vi "MGI RWA Get Type Info.vi"(8 "Error In":errorcluster, 11 "Variant":variant) -> (0 "Error Out":errorcluster, 2 "Name":string, 3 "Type Enum":T1)   [LabVIEW 2018]
doc: "Return information about the datatype stored in Variant.\nType Enum is the type of data\nName is the name of the data\nIf the data is defined by a Type Definition, HasTypedef is true and Typedef contains information about the Type Definition.\n\nNote: This VI is similar to vi.lib/Utility/VariantDataType/GetTypeInfo.vi, and produces the exact same results, but this VI is much faster for Waveform Types. (For 4000 Waveform type elements, this VI takes around 8000 ms and the vi.lib takes around 1600 ms. \n\nAuthored by Robert C. Mortensen\nsupport@mooregoodideas.com\nwww.mooregoodideas.com\n\nCopyright (c) 2010, Moore Good Ideas, Inc.\n\nAll rights reserved.\n\nRedistribution and use in source and binary forms, with or without modification, are permitted provided that the following conditions are met:\n\n * Redistributions of source code must retain the above copyright notice, this list of conditions and the following disclaimer.\n * Redistributions in binary form must reproduce the above copyright notice, this list of conditions and the following disclaimer in the documentation and/or other materials provided with the distribution.\n * Neither the name of Moore Good Ideas, Inc. nor the names of its contributors may be used to endorse or promote products derived from this software without specific prior written permission.\n\nTHIS SOFTWARE IS PROVIDED BY THE COPYRIGHT HOLDERS AND CONTRIBUTORS \"AS IS\" AND ANY EXPRESS OR IMPLIED WARRANTIES, INCLUDING, BUT NOT LIMITED TO, THE IMPLIED WARRANTIES OF MERCHANTABILITY AND FITNESS FOR A PARTICULAR PURPOSE ARE DISCLAIMED. IN NO EVENT SHALL THE COPYRIGHT OWNER OR CONTRIBUTORS BE LIABLE FOR ANY DIRECT, INDIRECT, INCIDENTAL, SPECIAL, EXEMPLARY, OR CONSEQUENTIAL DAMAGES (INCLUDING, BUT NOT LIMITED TO, PROCUREMENT OF SUBSTITUTE GOODS OR SERVICES; LOSS OF USE, DATA, OR PROFITS; OR BUSINESS INTERRUPTION) HOWEVER CAUSED AND ON ANY THEORY OF LIABILITY, WHETHER IN CONTRACT, STRICT LIABILITY, OR TORT (INCLUDING NEGLIGENCE OR OTHERWISE) ARISING IN ANY WAY OUT OF THE USE OF THIS SOFTWARE, EVEN IF ADVISED OF THE POSSIBILITY OF SUCH DAMAGE."
uses:
  Type.ctl
  TypedefInfo.ctl
  VariantType.lvlib
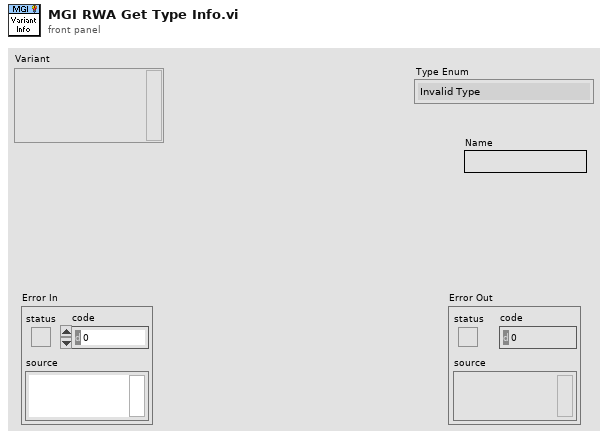
[diagram p1: front panel]
types:
  T1 = typedef "VariantType.lvlib/Type.ctl" = enum8{"Invalid Type", "Void", "I8", "I16", "I32", "I64", "U8", "U16", "U32", "U64", "Single Float", "Double Float", "Extended Float", "Single Complex", "Double Complex", "Extended Complex", "Enum U8", "Enum U16", "Enum U32", "Enum U64", "Single Float With Unit", "Double Float With Unit", "Extended Float With Unit", "Single Complex with Unit", "Double Complex with Unit", "Extended Complex with Unit", "Boolean", "String", "Path", "Picture", "Tag", "Array", "Cluster", "Variant", "LV Variant", "Waveform", "Timestamp", "Digital Waveform", "Digital Data", "ExpressData", "Refnum", "External Data", "VI", "Poly VI", "LabVIEW Class Instance", "Fixed Point"}
  T2 = typedef "VariantType.lvlib/TypedefInfo.ctl" = cluster{"Name":string, "Timestamp":u32}
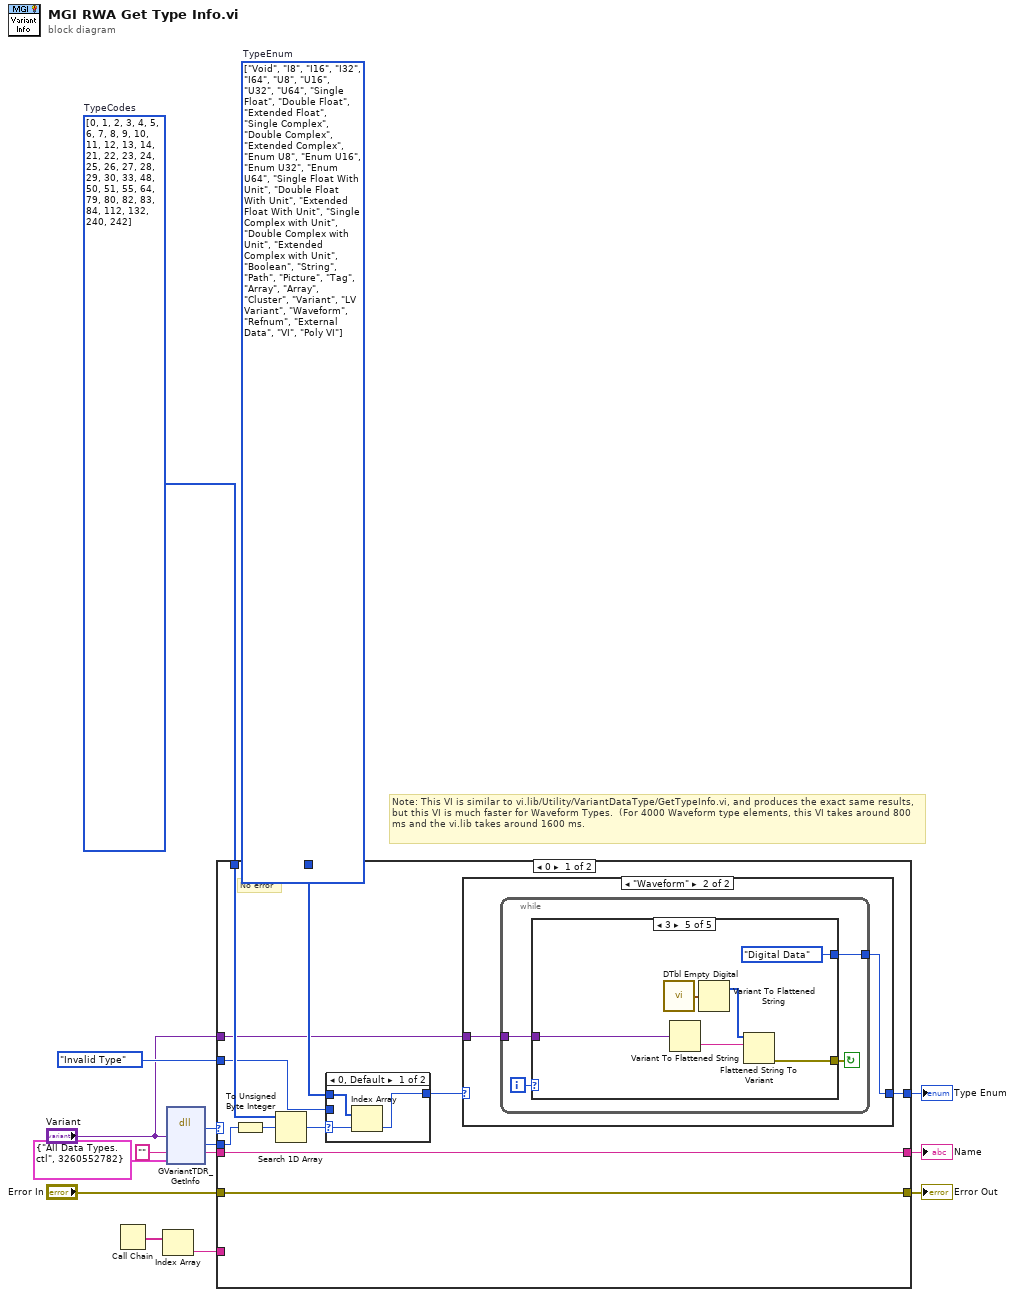
[diagram p0: block diagram]
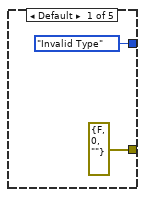
[diagram p3: hidden frame]
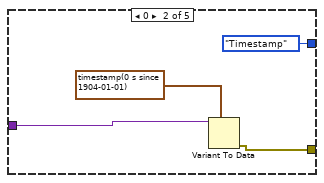
[diagram p4: hidden frame]
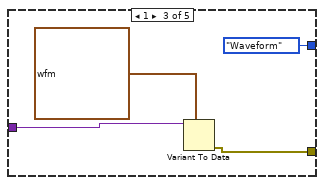
[diagram p5: hidden frame]
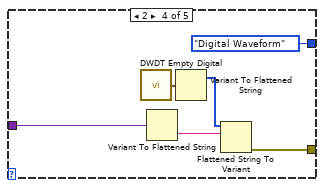
[diagram p6: hidden frame]
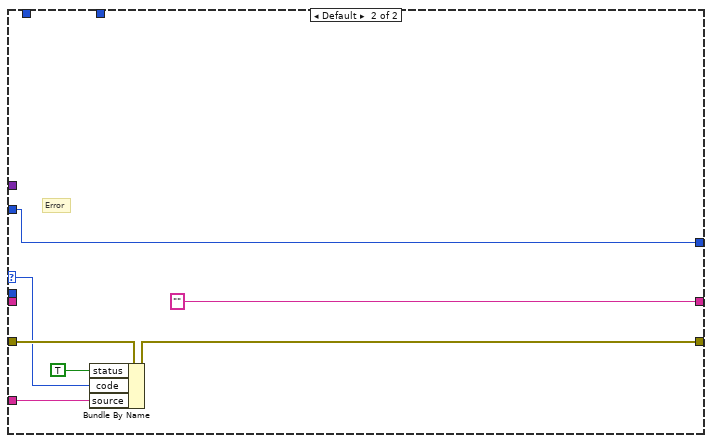
[diagram p8: hidden frame]
diagram:
  w10 = T1[] [enum."Void", enum."I8", enum."I16", enum."I32", enum."I64", enum."U8", enum."U16", enum."U32", enum."U64", enum."Single Float", enum."Double Float", enum."Extended Float", enum."Single Complex", enum."Double Complex", enum."Extended Complex", enum."Enum U8", enum."Enum U16", enum."Enum U32", enum."Enum U64", enum."Single Float With Unit", enum."Double Float With Unit", enum."Extended Float With Unit", enum."Single Complex with Unit", enum."Double Complex with Unit", enum."Extended Complex with Unit", enum."Boolean", enum."String", enum."Path", enum."Picture", enum."Tag", enum."Array", enum."Array", enum."Cluster", enum."Variant", enum."LV Variant", enum."Waveform", enum."Refnum", enum."External Data", enum."VI", enum."Poly VI"] items=["Invalid Type", "Void", "I8", "I16", "I32", "I64", "U8", "U16", "U32", "U64", "Single Float", "Double Float", "Extended Float", "Single Complex", "Double Complex", "Extended Complex", "Enum U8", "Enum U16", "Enum U32", "Enum U64", "Single Float With Unit", "Double Float With Unit", "Extended Float With Unit", "Single Complex with Unit", "Double Complex with Unit", "Extended Complex with Unit", "Boolean", "String", "Path", "Picture", "Tag", "Array", "Cluster", "Variant", "LV Variant", "Waveform", "Timestamp", "Digital Waveform", "Digital Data", "ExpressData", "Refnum", "External Data", "VI", "Poly VI", "LabVIEW Class Instance", "Fixed Point"]  # TypeEnum
  w12 = u8[] [0, 1, 2, 3, 4, 5, 6, 7, 8, 9, 10, 11, 12, 13, 14, 21, 22, 23, 24, 25, 26, 27, 28, 29, 30, 33, 48, 50, 51, 55, 64, 79, 80, 82, 83, 84, 112, 132, 240, 242]  # TypeCodes
  # "Note: This VI is similar to vi.lib/Utility/VariantDataType/GetTypeInfo.vi, and produces the exact same results, but this VI is much faster for Waveform Types.  (For 4000 Waveform type elements, this VI takes around 800 ms and the vi.lib takes around 1600 ms."
  n1 = Call Chain() -> (call chain=w8:string[])
  n2 = Index Array(array=w8) -> (element=w7:string)  [unwired: 1 in]
  n3 = dll-call lib="LabVIEW" fn="GVariantTDR_GetInfo"("Variant"="Variant", "name"="", "TypedefInfo"=T2 {"Name"="All Data Types.ctl", "Timestamp"=3260552782}) -> (w6:i32, "typeCode"=w5:i16, "name"=w4:string)  [unwired: 6 in, 2 out]
  n4 = case shown="0" w6 {
    selector: w6 -> [_ w63]
    tunnel: w5 -> [w25 _]
    tunnel: w4 -> [w26 _]
    tunnel: [w18 w61] -> w2
    tunnel: [w26 "" ("name")] -> w15
    tunnel: "Error In" -> [w16 w65]
    tunnel: [w16 w64] -> w13
    tunnel: Type."Invalid Type" ("Type Enum 2") -> [w20 w61]
    tunnel: w12 -> [w22 _]
    tunnel: w10 -> [w21 _]
    tunnel: w7 -> [_ w60]
    tunnel: "Variant" -> [w17 _]
    frame 0 {
      # "No error"
      n5 = To Unsigned Byte Integer(number=w25) -> (unsigned 8bit integer=w24:u8)
      n6 = Search 1D Array(1D array=w22, element=w24) -> (index of element=w23:i32)  [unwired: 1 in]
      n7 = case shown="0, Default" w23 {
        selector: w23 -> [w58 _]
        tunnel: [w57 w59] -> w19
        tunnel: w21 -> [w56 _]
        tunnel: w20 -> [_ w59]
        frame 0, Default {
          n8 = Index Array(array=w56, index=w58) -> (element=w57:T1)
        }
        frame -1 {
        }
      }
      n9 = case shown="\"Waveform\"" w19 {
        selector: w19 -> [w27 _]
        tunnel: [w27 w28] -> w18
        tunnel: w17 -> [_ w29]
        frame Default {
        }
        frame "Waveform" {
          n10 = while {
            tunnel: w29 -> [w32]
            tunnel: [w30] -> w28
            i -> [w33]
            stop <- w31 continue-if-true
            n11 = case shown="3" w33 {
              tunnel: w32 -> [_ w37 w42 w49 w55]
              tunnel: [errorcluster {"status"=FALSE, "code"=0, "source"=""} ("error out") w36 w40 w46 w52] -> w31
              tunnel: [Type."Invalid Type" ("Type Enum") Type."Timestamp" ("Type Enum") Type."Waveform" ("Type Enum") Type."Digital Waveform" ("Type Enum") Type."Digital Data" ("Type Enum")] -> w30
              frame Default {
              }
              frame 0 {
                n12 = Variant To Data(type=timestamp(0 s since 1904-01-01), Variant=w37) -> (error out=w36:errorcluster)  [unwired: 1 in, 1 out]
              }
              frame 1 {
                n13 = Variant To Data(type=waveform(dbl) {"t0"=timestamp(0 s since 1904-01-01), "dt"=0.0, "Y"=[]} ("Waveform 2"), Variant=w42) -> (error out=w40:errorcluster)  [unwired: 1 in, 1 out]
              }
              frame 2 {
                n14 = call "DWDT Empty Digital.vi"() -> ("digital waveform out"=w44:digitalwaveform)  [unwired: 5 in]
                n15 = Variant To Flattened String(Variant=w49) -> (data string=w47:string)  [unwired: 1 out]
                n16 = Variant To Flattened String(Variant=w44) -> (1:w48:i16[])  [unwired: 1 out]
                n17 = Flattened String To Variant(6:w47, 7:w48) -> (0:w46:errorcluster)  [unwired: 1 in, 1 out]
              }
              frame 3 {
                n18 = call "DTbl Empty Digital.vi"() -> ("digital data"=w50:digitaldata)  [unwired: 5 in]
                n19 = Variant To Flattened String(Variant=w55) -> (data string=w53:string)  [unwired: 1 out]
                n20 = Variant To Flattened String(Variant=w50) -> (1:w54:i16[])  [unwired: 1 out]
                n21 = Flattened String To Variant(6:w53, 7:w54) -> (0:w52:errorcluster)  [unwired: 1 in, 1 out]
              }
            }
          }
        }
      }
    }
    frame Default {
      # "Error"
      n22 = Bundle By Name(cluster=w65, "status"=TRUE, "code"=w63, "source"=w60) -> (w64:errorcluster)
    }
  }
  "Name" <- w15
  "Error Out" <- w13
  "Type Enum" <- w2
